vi "Input Data.vi"() -> ()   [LabVIEW 2013]
uses:
  qwtb_lvlib/TD Quantity.ctl
  globals.vi
  <vilib>/Utility/xml.llb/Write to XML File(string).vi
  <vilib>/Utility/xml.llb/Read From XML File(string).vi
panel:
  in  "Q list signaling":i32
  in  "close":bool
  in  "Selected Quantity":T1={"Name"="", "Value"=[[1.0]], "Uncertainty"=[[1.0]], "Degrees of\nFreedom"=[[10.0]], "Correlation"=[[10.0]], "Randomized uncertainty"=[[10.0]]}
  in  "load Q":bool
  in  "save Q":bool
  in  "Q list":i32(listbox) caption="Input Quantities"
  in  "remove Q":bool
  in  "add Q":bool
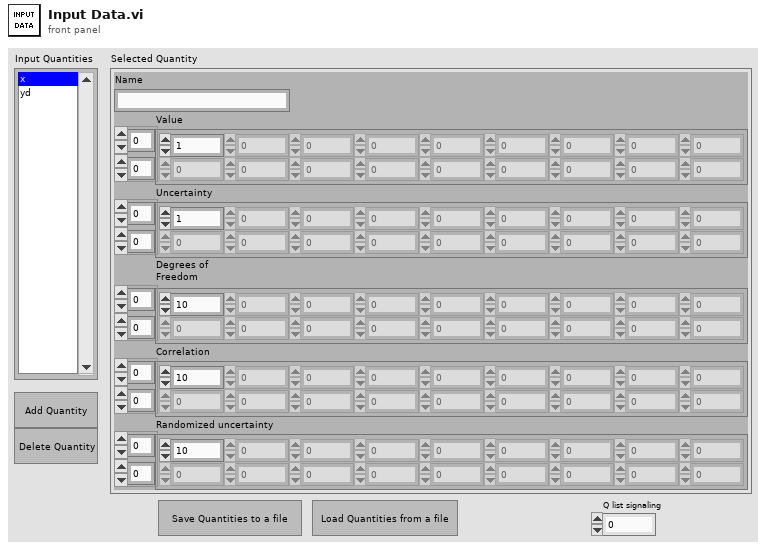
[diagram p1: front panel]
types:
  T1 = typedef "TD Quantity.ctl" = cluster{"Name":string, "Value":dbl[][], "Uncertainty":dbl[][], "Degrees of\nFreedom":dbl[][], "Correlation":dbl[][], "Randomized uncertainty":dbl[][]}
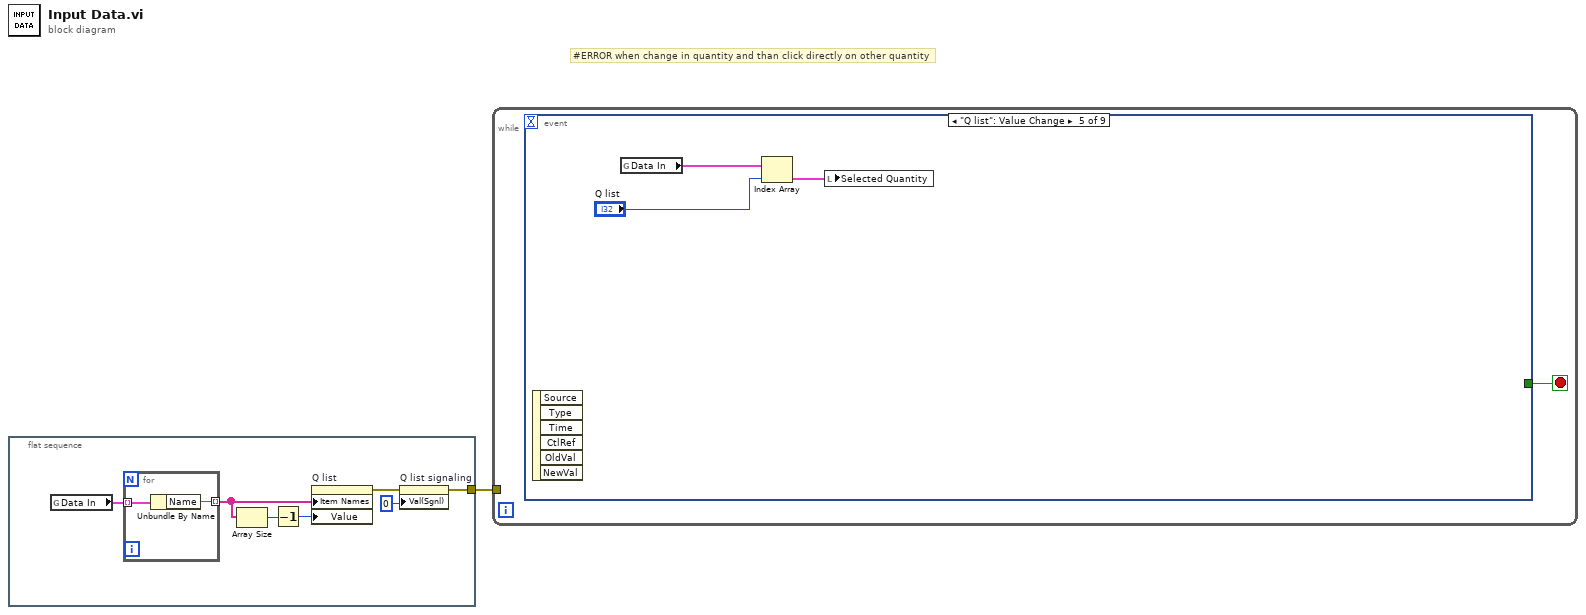
[diagram p0: block diagram]
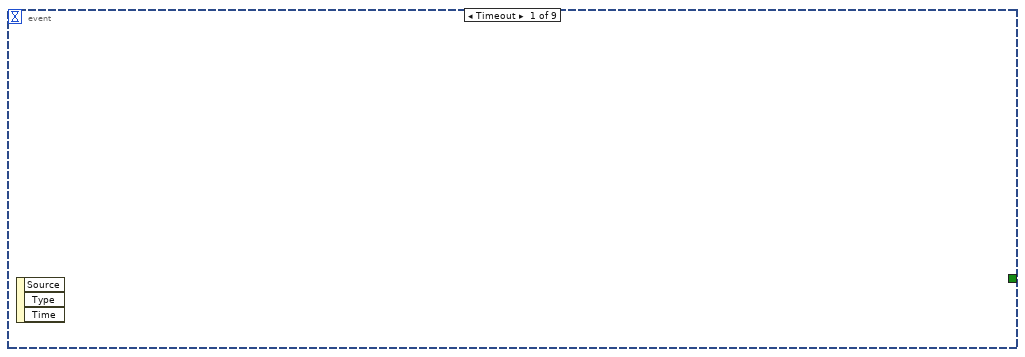
[diagram p2: hidden frame]
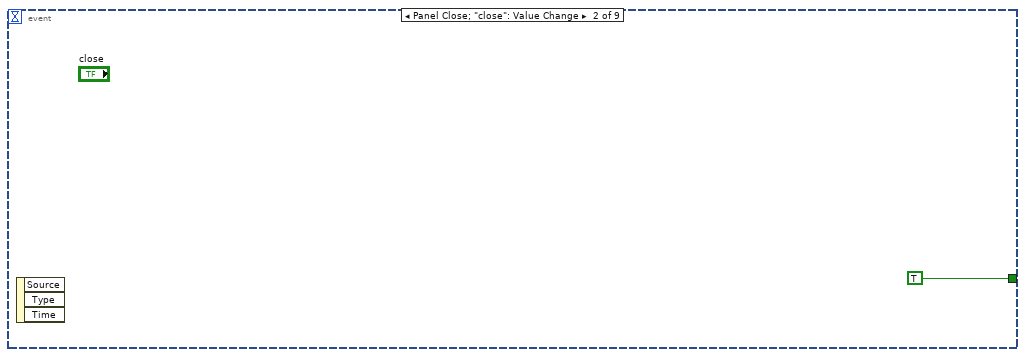
[diagram p3: hidden frame]
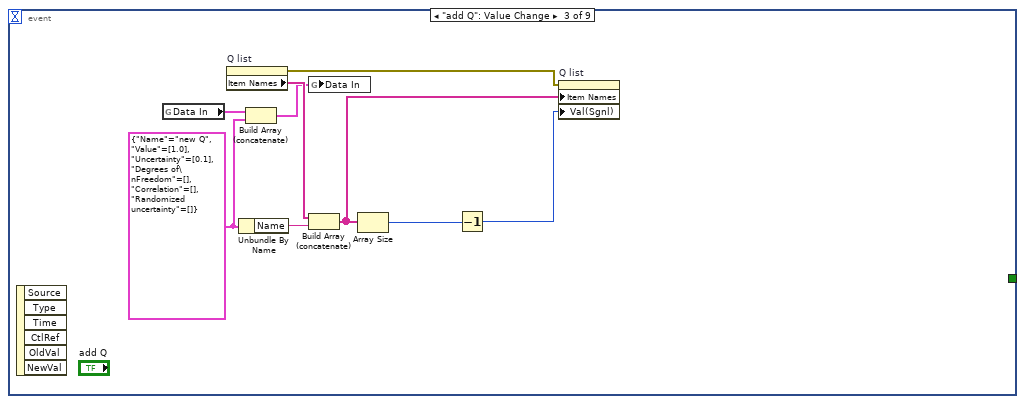
[diagram p4: hidden frame]
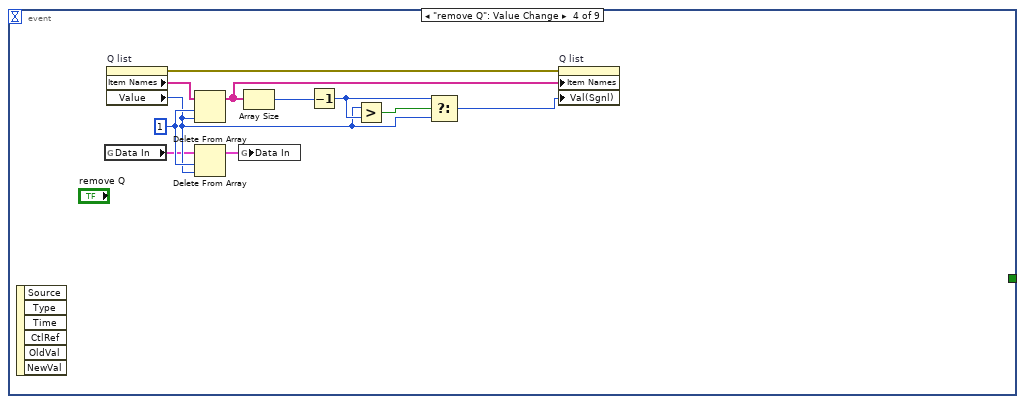
[diagram p5: hidden frame]
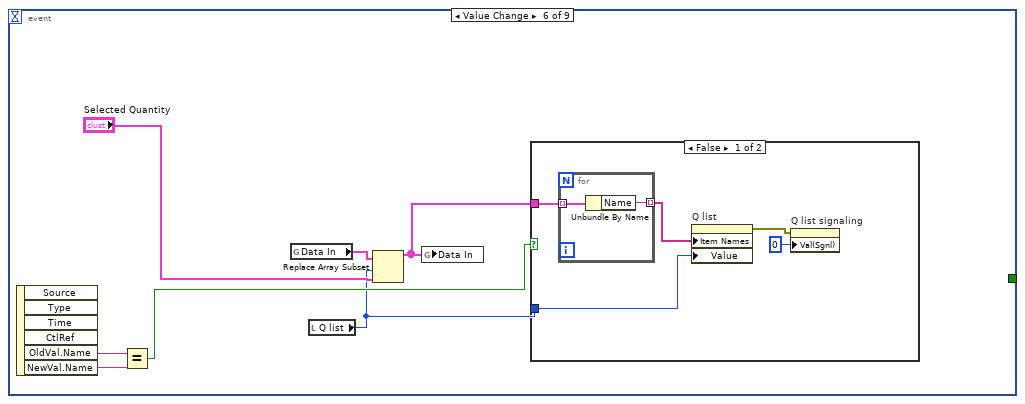
[diagram p6: hidden frame]
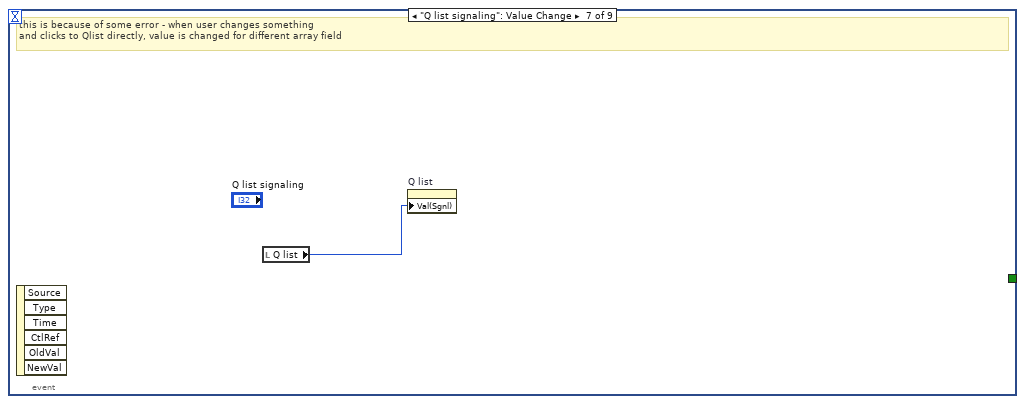
[diagram p8: hidden frame]
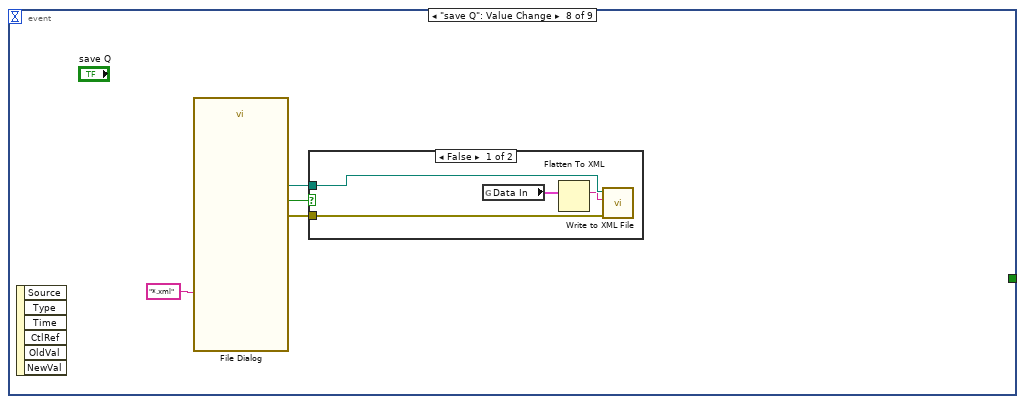
[diagram p9: hidden frame]
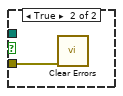
[diagram p10: hidden frame]
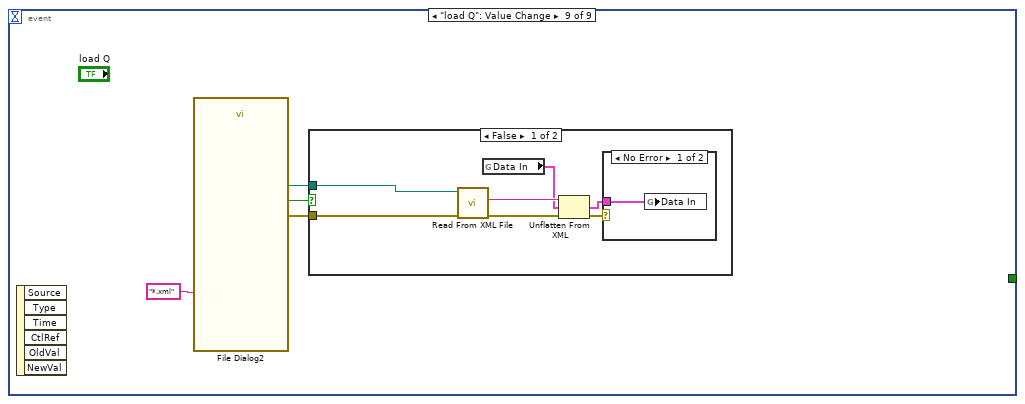
[diagram p11: hidden frame]
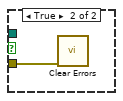
[diagram p13: hidden frame]
diagram:
  # "#ERROR when change in quantity and than click directly on other quantity"
  n1 = flat-sequence {
    tunnel: [w3] -> w1
    frame #0 {
      n2 = global read "globals.vi" "Data In"() -> (w7:T1[])
      n3 = for {
        tunnel: [w10] -> w8 mode=indexing
        tunnel: w7 -> [w9] mode=indexing
        n4 = Unbundle By Name(w9) -> ("Name"=w10:string)
      }
      n5 = Array Size(array=w8) -> (size(s)=w6:i32)
      n6 = Decrement(x=w6) -> (x-1=w5:i32)
      n7 = property on="Q list" class="LstBox (strict)"("Item Names"=w8, "Value"=w5) -> (error out=w4:errorcluster)  [unwired: 2 in, 1 out]
      n8 = property on="Q list signaling" class="DigNum (strict)"(error in=w4, "Val(Sgnl)"=0 ("Value (Signaling)")) -> (error out=w3:errorcluster)  [unwired: 1 in, 1 out]
    }
  }
  n9 = while {
    tunnel: w1 -> [_]
    stop <- w11 stop-if-true
    n10 = event shown="[4] \"Q list\": Value Change" {
      selector: _ -> [_ _ _ _ _ _ _ _ _]
      dyn-events: _ -> [_ _ _ _ _ _ _ _ _]
      timeout: _ -> [_ _ _ _ _ _ _ _ _]
      tunnel: [_ TRUE _ _ _ _ _ _ _] -> w11
      event Timeout {
        n11 = event-data() -> ()  [unwired: 1 in, 3 out]
      }
      event Panel Close; "close": Value Change {
        n12 = event-data() -> ()  [unwired: 1 in, 3 out]
      }
      event "add Q": Value Change {
        w15 = T1 {"Name"="new Q", "Value"=[[1.0]], "Uncertainty"=[[0.1]], "Degrees of\nFreedom"=[], "Correlation"=[], "Randomized uncertainty"=[]} ("Quantity")
        n13 = event-data() -> ()  [unwired: 1 in, 6 out]
        n14 = global read "globals.vi" "Data In"() -> (w14:T1[])
        n15 = property on="Q list" class="LstBox (strict)"() -> (error out=w20:errorcluster, "Item Names"=w21:string[])  [unwired: 2 in, 1 out]
        n16 = Unbundle By Name(w15) -> ("Name"=w16:string)
        n17 = Build Array (concatenate)(w14, w15) -> (w13:T1[])
        n18 = global write "globals.vi" "Data In"(w13) -> ()
        n19 = Build Array (concatenate)(w21, w16) -> (w19:string[])
        n20 = Array Size(array=w19) -> (size(s)=w18:i32)
        n21 = Decrement(x=w18) -> (x-1=w17:i32)
        n22 = property on="Q list" class="LstBox (strict)"(error in=w20, "Item Names"=w19, "Val(Sgnl)"=w17) -> ()  [unwired: 1 in, 2 out]
      }
      event "remove Q": Value Change {
        w25 = 1 ("length")
        n23 = event-data() -> ()  [unwired: 1 in, 6 out]
        n24 = global read "globals.vi" "Data In"() -> (w23:T1[])
        n25 = property on="Q list" class="LstBox (strict)"() -> (error out=w32:errorcluster, "Item Names"=w31:string[], "Value"=w24:i32)  [unwired: 2 in, 1 out]
        n26 = Delete From Array(array=w31, length=w25, index=w24) -> (array with subset deleted=w30:string[])  [unwired: 1 out]
        n27 = Delete From Array(array=w23, length=w25, index=w24) -> (array with subset deleted=w22:T1[])  [unwired: 1 out]
        n28 = global write "globals.vi" "Data In"(w22) -> ()
        n29 = Array Size(array=w30) -> (size(s)=w29:i32)
        n30 = Decrement(x=w29) -> (x-1=w27:i32)
        n31 = Greater?(x=w24, y=w27) -> (0:w28:bool)
        n32 = Select(t=w27, s=w28, f=w24) -> (s? t:f=w26:i32)
        n33 = property on="Q list" class="LstBox (strict)"(error in=w32, "Item Names"=w30, "Val(Sgnl)"=w26) -> ()  [unwired: 1 in, 2 out]
      }
      event "Q list": Value Change {
        n34 = event-data() -> ()  [unwired: 1 in, 6 out]
        n35 = global read "globals.vi" "Data In"() -> (w35:T1[])
        n36 = Index Array(array=w35, index="Q list") -> (element=w33:T1)
        n37 = local write "Selected Quantity"(w33) -> ()
      }
      event Value Change {
        n38 = event-data() -> ("OldVal.Name"=w42:string, "NewVal.Name"=w41:string)  [unwired: 1 in, 4 out]
        n39 = Equal?(x=w42, y=w41) -> (x = y?=w37:bool)
        n40 = global read "globals.vi" "Data In"() -> (w39:T1[])
        n41 = local read "Q list"() -> (w36:i32)
        n42 = Replace Array Subset(array=w39, new element="Selected Quantity", index=w36) -> (w38:T1[])
        n43 = global write "globals.vi" "Data In"(w38) -> ()
        n44 = case shown="False" w37 {
          tunnel: w38 -> [w46 _]
          tunnel: w36 -> [w45 _]
          frame False {
            n45 = for {
              tunnel: [w49] -> w47 mode=indexing
              tunnel: w46 -> [w48] mode=indexing
              n46 = Unbundle By Name(w48) -> ("Name"=w49:string)
            }
            n47 = property on="Q list" class="LstBox (strict)"("Item Names"=w47, "Value"=w45) -> (error out=w44:errorcluster)  [unwired: 2 in, 1 out]
            n48 = property on="Q list signaling" class="DigNum (strict)"(error in=w44, "Val(Sgnl)"=0 ("Value (Signaling)")) -> ()  [unwired: 1 in, 2 out]
          }
          frame True {
          }
        }
      }
      event "Q list signaling": Value Change {
        # "this is because of some error - when user changes something\nand clicks to Qlist directly, value is changed for different array field"
        n49 = event-data() -> ()  [unwired: 1 in, 6 out]
        n50 = local read "Q list"() -> (w50:i32)
        n51 = property on="Q list" class="LstBox (strict)"("Val(Sgnl)"=w50) -> ()  [unwired: 2 in, 2 out]
      }
      event "save Q": Value Change {
        n52 = event-data() -> ()  [unwired: 1 in, 6 out]
        n53 = call "File Dialog"("pattern (all files)"="*.xml") -> ("selected path"=w54:path, "cancelled"=w52:bool, "error out"=w53:errorcluster)  [unwired: 11 in, 1 out]
        n54 = case shown="False" w52 {
          tunnel: w53 -> [w57 w59]
          tunnel: w54 -> [w58 _]
          frame False {
            n55 = global read "globals.vi" "Data In"() -> (w55:T1[])
            n56 = Flatten To XML(anything=w55) -> (xml string=w56:string)
            n57 = call-poly <vilib>:"Write to XML File.vi"("error in (no error)"=w57, "XML Input"=w56, "XML File Path"=w58) -> ()  [unwired: 6 in, 3 out]
          }
          frame True {
            n58 = call <vilib>:"Clear Errors.vi"("error in (no error)"=w59) -> ()  [unwired: 6 in, 1 out]
          }
        }
      }
      event "load Q": Value Change {
        n59 = event-data() -> ()  [unwired: 1 in, 6 out]
        n60 = call "File Dialog2"("pattern (all files)"="*.xml") -> ("selected path"=w63:path, "cancelled"=w61:bool, "error out"=w62:errorcluster)  [unwired: 11 in, 1 out]
        n61 = case shown="False" w61 {
          tunnel: w62 -> [w69 w72]
          tunnel: w63 -> [w70 _]
          frame False {
            n62 = call-poly <vilib>:"Read From XML File.vi"("error in (no error)"=w69, "XML File Path"=w70) -> ("error out"=w67:errorcluster, "XML Elements"=w68:string)  [unwired: 7 in, 1 out]
            n63 = global read "globals.vi" "Data In"() -> (w64:T1[])
            n64 = Unflatten From XML(xml string=w68, type=w64, error in (no error)=w67) -> (value=w65:T1[], error out=w66:errorcluster)
            n65 = case shown="No Error" w66 {
              tunnel: w65 -> [w71 _]
              frame No Error {
                n66 = global write "globals.vi" "Data In"(w71) -> ()
              }
              frame Error {
              }
            }
          }
          frame True {
            n67 = call <vilib>:"Clear Errors.vi"("error in (no error)"=w72) -> ()  [unwired: 6 in, 1 out]
          }
        }
      }
    }
  }
